vi "Test Load 16-bit PNG (Path).vi"(8 "error in (no error)":errorcluster) -> (0 "error out":errorcluster, 3 "Pass?":bool)   [LabVIEW 2020]
uses:
  9f3bbfbf-8e98-45eb-a787-ef2e68e6fd36.vi
  G-Image/Image IO/Polymorphic VIs/Load Image (16-bit) (Path).vi
  G-Image/G-Image.lvlib
panel:
  out "Array":cluster{string, "new picture":picture}[](array[cluster])
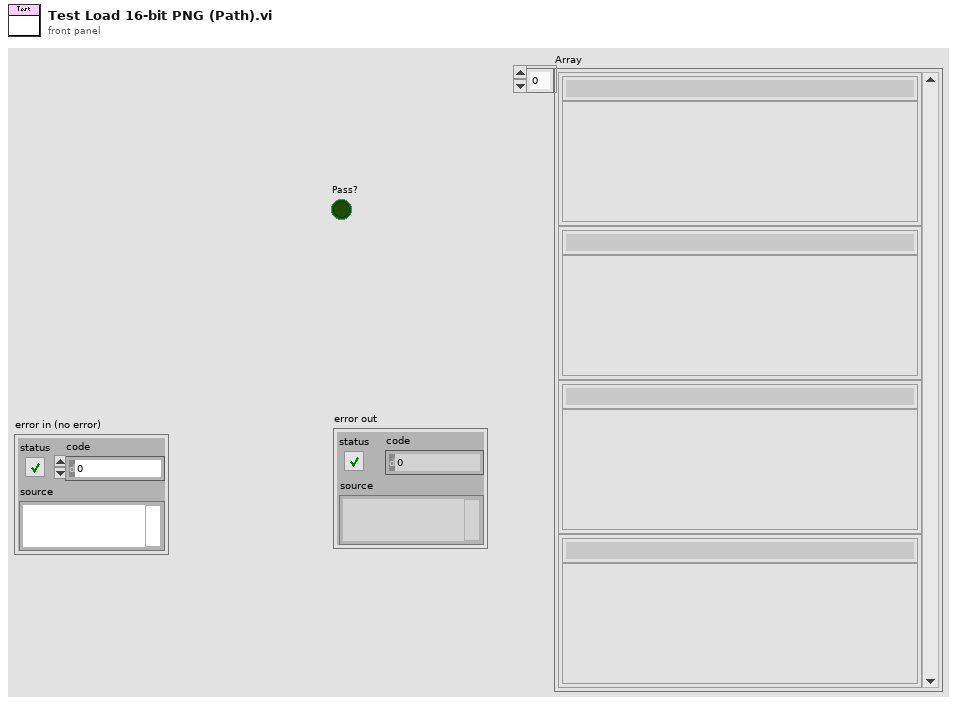
[diagram p1: front panel]
types:
  T1 = typedef "G-Image.lvlib/Image 16-bit.ctl" = cluster{"image type":i32, "image depth":i32, "image":u16[], "mask":u8[], "colors":u32[], "Rectangle":cluster{"left":i16, "top":i16, "right":i16, "bottom":i16}}
  T2 = typedef "imagedata.ctl" = cluster{"image type":i32, "image depth":i32, "image":u8[], "mask":u8[], "colors":u32[], "Rectangle":cluster{"left":i16, "top":i16, "right":i16, "bottom":i16}}
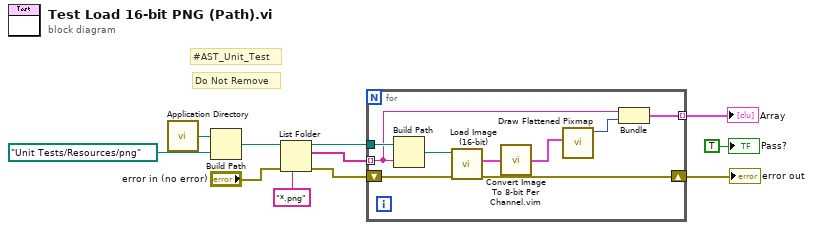
[diagram p0: block diagram]
diagram:
  # "Do Not Remove"
  # "#AST_Unit_Test"
  n1 = call <vilib>:"Application Directory.vi"() -> ("Application Directory"=w11:path)
  n2 = Build Path(base path=w11, name or relative path=path "Unit Tests/Resources/png" ("Path")) -> (appended path=w9:path)
  n3 = List Folder(path=w9, pattern="*.png", error in="error in (no error)") -> (path out=w7:path, filenames=w6:string[], error out=w4:errorcluster)  [unwired: 1 in, 1 out]
  n4 = for {
    tunnel: w7 -> [w20]
    tunnel: w6 -> [w14] mode=indexing
    shift-right: [w17] -> w3
    shift-left: w4 -> [w18]
    tunnel: [w13] -> w2 mode=indexing
    n5 = Build Path(base path=w20, name or relative path=w14) -> (appended path=w19:path)
    n6 = call-poly "Load Image (16-bit).vi"("error in (no error)"=w18, "Path In"=w19) -> ("error out"=w17:errorcluster, "Image (16-bit)"=w16:T1)  [unwired: 7 in, 1 out]
    n7 = call "Convert Image To 8-bit Per Channel.vim"("Image (16-bit)"=w16) -> ("Image"=w12:T2)
    n8 = call <vilib>:"Draw Flattened Pixmap.vi"("image data"=w12) -> ("new picture"=w15:picture)  [unwired: 8 in]
    n9 = Bundle(w14, "new picture"=w15) -> (w13:cluster{string, "new picture":picture})  [unwired: 1 in]
  }
  "error out" <- w3
  "Array" <- w2
  "Pass?" <- TRUE ("Pass?")
